vi "Write String.vi"(10 "string":string) -> (3 "String Without Equals":refnum<class "String Without Equals.lvclass">)   [LabVIEW 2023, in "String Without Equals.lvclass"]
uses:
  String Without Equals.lvclass
  String Without Equals.lvclass/String Without Equals.ctl
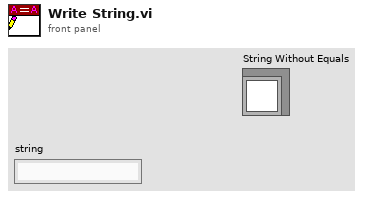
[diagram p1: front panel]
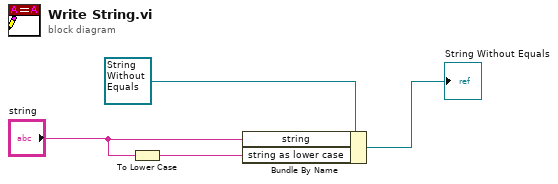
[diagram p0: block diagram]
diagram:
  n1 = To Lower Case(string="string") -> (all lower case string=w1:string)
  n2 = Bundle By Name(cluster=refnum<class "String Without Equals.lvclass"> refnum ("String Without Equals in"), "string"="string", "string as lower case"=w1) -> (→"String Without Equals":refnum<class "String Without Equals.lvclass">)
